vi "CLD 2  Elapsed Time Express with pause Solution.vi"() -> ()   [LabVIEW 2009]
doc: "This VI demonstrates one implementation of adding pause capability to the Elapsed Time Express VI. This method uses the 'set start time' input and tracks real time in order to imitate a pause.\n\nAnother Method would be to keep track of the elapsed time and change the time target when timing continues. That method is more cumbersome and presents additional overhead if the VI must display the original time target.\n\nThe Pause \"Time Slipper\" case structure description of operation.\n\nFalse case: No Pause, standard timer\n\nThe present time is passed to the recirculate shift register. The recirculate time is used to know when the timer last was not in pause and it will be used to find the delta time when the pause is removed. Not used as long as the pause is false.\n\nThe Start Time is used and passed along. Once the Time Has Elapsed is TRUE, then pass the new present time to the start time.\n\nTrue Case: Pause Pressed\nCalculate the difference of time between the last time when pause was FALSE (Recirculate time) and the current time. Add this delta time (Dwell time in pause) to the start time of the timer, i.e. slide the start time.\n\nThe recirculate time shift register is still the present time."
panel:
  out "Elapsed Time (s)":dbl format="%#.1g"
  out "Time Has Elapsed":bool
  in  "Auto Reset":bool
  in  "Pause Button":bool
  in  "Reset Button":bool
  in  "Stop VI":bool
  out "error out":errorcluster
  in  "Error In":errorcluster
  in  "Time Target (s)":dbl
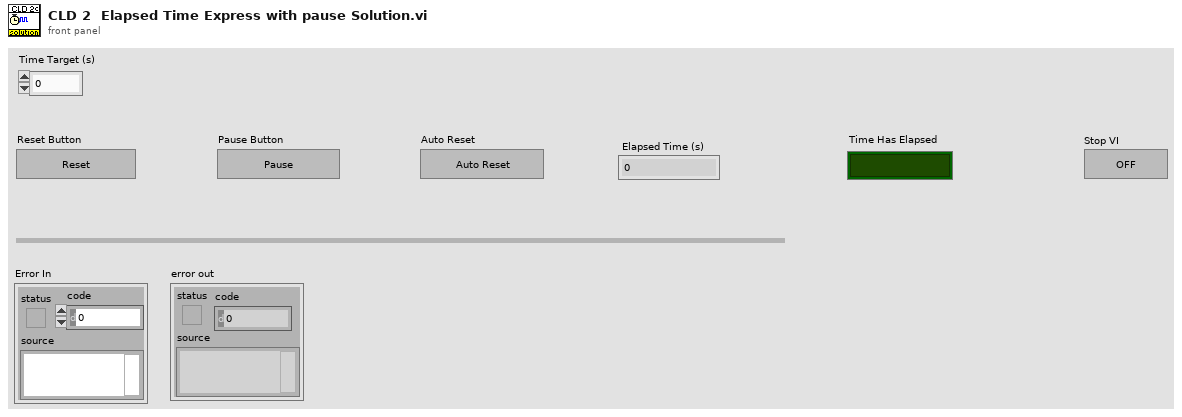
[diagram p1: front panel]
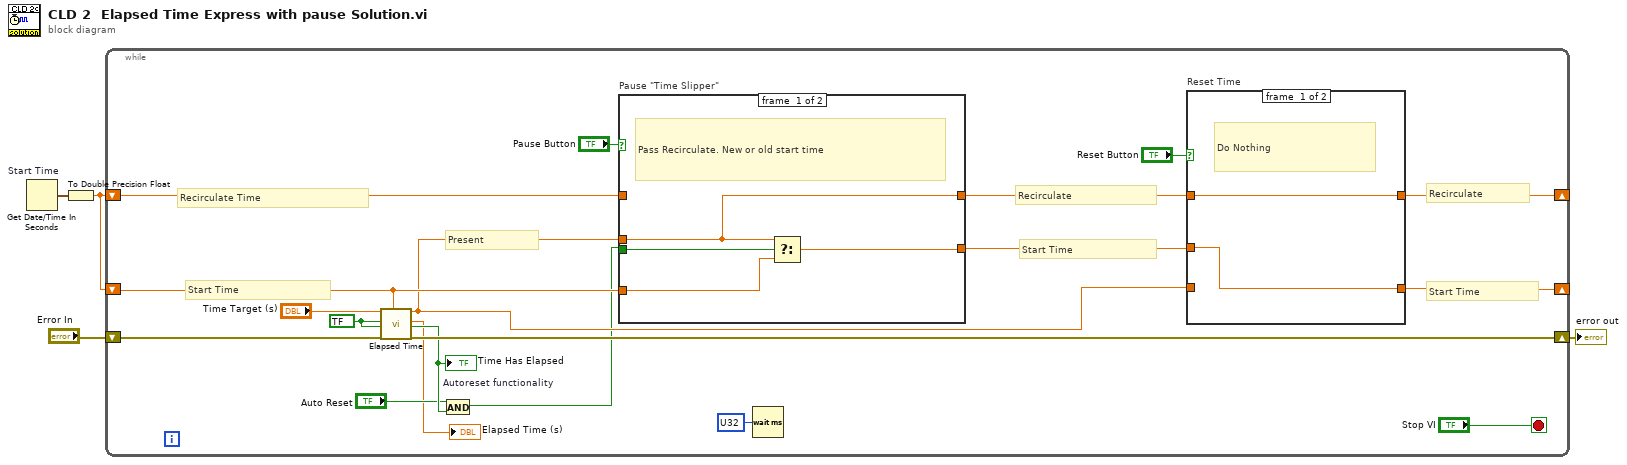
[diagram p0: block diagram]
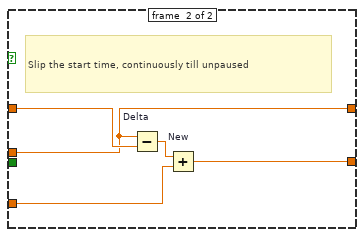
[diagram p3: hidden frame]
diagram:
  n1 = Get Date/Time In Seconds "Start Time"() -> (seconds since 1Jan1904=w2:timestamp)
  n2 = To Double Precision Float(number=w2) -> (double precision float=w1:dbl)
  n3 = while {
    shift-right: [w11] -> _
    shift-left: w1 -> [w20]
    shift-right: [w17] -> w3
    shift-left: "Error In" -> [w18]
    shift-right: [w13] -> _
    shift-left: w1 -> [w16]
    stop <- "Stop VI" stop-if-true
    w8 = bool ? ("Reset")
    # "Present"
    # "Start Time"
    # "Recirculate Time"
    # "Recirculate"
    # "Recirculate"
    # "Start Time"
    # "Start Time"
    n4 = call "Elapsed Time"("Time Target (s)"="Time Target (s)", "Reset"=w8, "Auto Reset"=w8, "error in (no error)"=w18, "Set Start Time (s)"=w20) -> ("Present (s)"=w10:dbl, "Elapsed Time (s)"=→"Elapsed Time (s)":dbl, "Time has Elapsed"=w9:bool, "error out"=w17:errorcluster)  [unwired: 7 in, 4 out]
    "Time Has Elapsed" <- w9
    n5 = And "Autoreset functionality"(x="Auto Reset", y=w9) -> (x .and. y?=w7:bool)
    n6 = case "Pause \"Time Slipper\"" shown="True" "Pause Button" {
      tunnel: w7 -> [w30 _]
      tunnel: w10 -> [w27 w31]
      tunnel: [w29 w33] -> w12
      tunnel: w20 -> [w28 w32]
      tunnel: [w27 w31] -> w14
      tunnel: w16 -> [_ w34]
      frame #0 {
        # "Pass Recirculate. New or old start time"
        n7 = Select(t=w27, s=w30, f=w28) -> (s? t:f=w29:dbl)
      }
      frame #1 {
        # "Slip the start time, continuously till unpaused"
        n8 = Subtract "Delta"(x=w31, y=w34) -> (x-y=w35:dbl)
        n9 = Add "New"(x=w35, y=w32) -> (x+y=w33:dbl)
      }
    }
    n10 = Wait (ms)(milliseconds to wait=u32 ?) -> ()  [unwired: 1 out]
    n11 = case "Reset Time" shown="True" "Reset Button" {
      tunnel: [w25 w26] -> w13
      tunnel: w14 -> [w25 _]
      tunnel: [w24 w26] -> w11
      tunnel: w12 -> [w24 _]
      tunnel: w10 -> [_ w26]
      frame #0 {
        # "Do Nothing"
      }
      frame #1 {
        # "Set Both times the same"
      }
    }
  }
  "error out" <- w3
